vi "get operating mode.vi"(8 "error in (no error)":errorcluster, 11 "Cobolt in":refnum<class "Cobolt.lvclass">) -> (0 "error out":errorcluster, 3 "Cobolt out":refnum<class "Cobolt.lvclass">)   [LabVIEW 2012, in "Cobolt.lvclass"]
uses:
  Cobolt.lvclass
  CoboltLaserDrivers_Public_LV2012/CoboltLaser_Controls/ExpectedResponseType.ctl
  Cobolt.lvclass/Cobolt.ctl
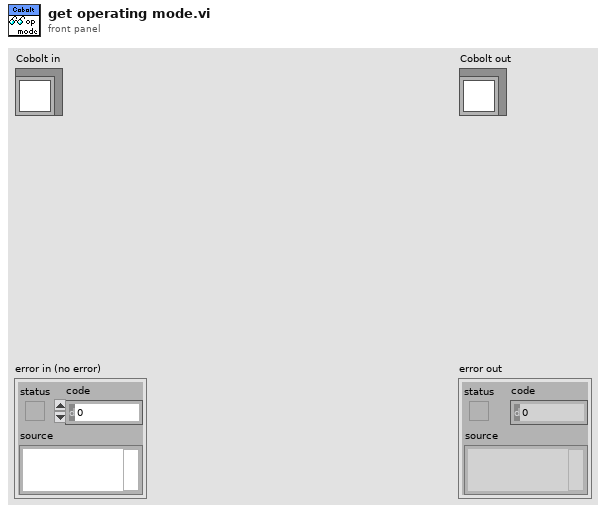
[diagram p1: front panel]
types:
  T1 = typedef "Cobolt.lvclass/ExpectedResponseType.ctl" = u16
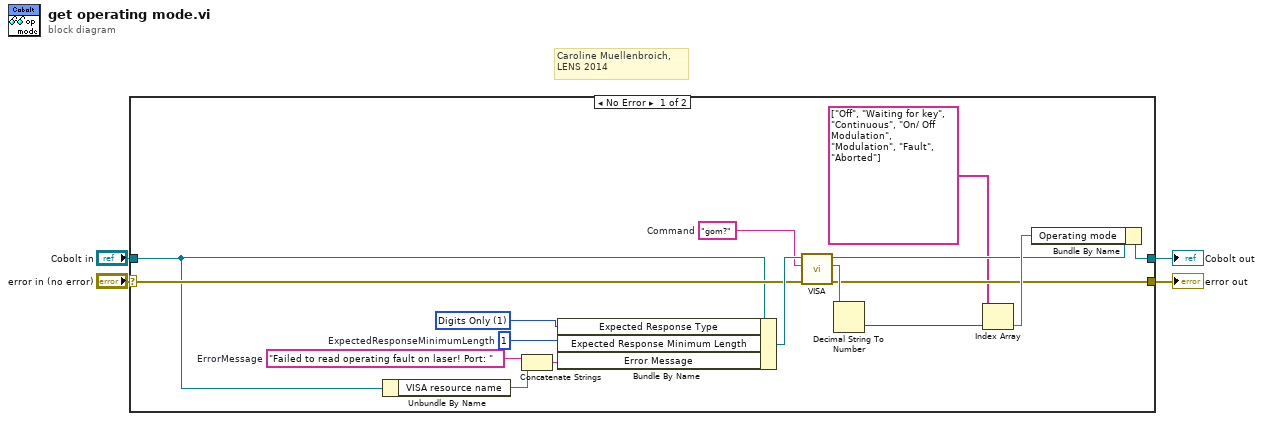
[diagram p0: block diagram]
diagram:
  # "Caroline Muellenbroich, \nLENS 2014"
  n1 = case shown="No Error" "error in (no error)" {
    selector: "error in (no error)" -> [w9 w22]
    tunnel: [w8 w22] -> w3
    tunnel: [w6 w21] -> w1
    tunnel: "Cobolt in" -> [w7 w21]
    frame No Error {
      w17 = T1 1 items=["Any", "Digits Only", "Non-Digits Only"] ("ExpectedResponseType")
      w13 = 1  # ExpectedResponseMinimumLength
      w15 = "Failed to read operating fault on laser! Port: "  # ErrorMessage
      w11 = "gom?"  # Command
      n2 = Unbundle By Name(w7) -> ("VISA resource name"=w14:string)
      n3 = Concatenate Strings(w15, w14) -> (w16:string)
      n4 = Bundle By Name(cluster=w7, "Expected Response Type"=w17, "Expected Response Minimum Length"=w13, "Error Message"=w16) -> (w12:refnum<class "Cobolt.lvclass">)
      n5 = call-dynamic "VISA.vi"("error in (no error)"=w9, "string to write"=w11, "Cobolt in"=w12) -> ("error out"=w8:errorcluster, "buffer out"=w18:string, "Cobolt out"=w10:refnum<class "Cobolt.lvclass">)  [unwired: 6 in]
      n6 = Decimal String To Number(string=w18) -> (number=w19:i32)  [unwired: 2 in, 1 out]
      n7 = Index Array(array=string[] ["Off", "Waiting for key", "Continuous", "On/ Off Modulation", "Modulation", "Fault", "Aborted"], index=w19) -> (element=w20:string)
      n8 = Bundle By Name(cluster=w10, "Operating mode"=w20) -> (w6:refnum<class "Cobolt.lvclass">)
    }
    frame Error {
    }
  }
  "error out" <- w3
  "Cobolt out" <- w1
